vi "SOL Instruments Camera.vi"() -> ()   [LabVIEW 2015]
doc: "Example VI that demonstrates all library features."
uses:
  PL SOL Instruments Camera.lvclass
panel:
  in  "port":u16=17017
  in  "address":string="192.168.240.181"
  out "SOL Camera":refnum<class "PL SOL Instruments Camera.lvclass">
  out "error":errorcluster
  in  "stop":bool
  in  "Tab Control":enum32{"Main", "Parameters", "Info"}(tab)
  out "graph":u16[](graph)
  in  "run once":bool
  in  "run":bool
  in  "offset":dbl=-30.59628543499511 format="%#_3g"
  in  "gain":dbl=1.6 format="%#_3g"
  in  "camera parameters":T1={"number of regions"=1, "readout rate, kHz"=1000, "actual readout rate, kHz"=0, "bits per pixel"=4, "synchronization mode"=0, "OUT1 mode"=0, "OUT2 mode"=0, "exposure time, s"=0.001, "delay before exposure, s"=1e-06, "delay after exposure, s"=1e-06, "delay between exposures, s"=1e-06, "CCD mode"=2, "CCD advanced mode"=0, "X read mode"=0, "Y read mode"=1, "prechanrge bus"=0, "options"={"x averaging"=FALSE, "x subsampling"=FALSE, "y subsampling"=FALSE, "y averaging"=FALSE}, "nondestructive frame delays, s"=[1e-06, 1e-06, 1e-06, 1e-06, 1e-06, 1e-06, 1e-06, 1e-06], "double slope reset time, s"=1e-06, "DAC"=32, "gamma correction"=0} {"double slope reset time, s" format="%#_6p"; "nondestructive frame delays, s" format="%#_3p"; "prechanrge bus" items=["no", "yes"]; "Y read mode" items=["forward", "backward"]; "X read mode" items=["forward", "backward"]; "CCD advanced mode" items=["none", "nondestructive", "double slope"]; "CCD mode" items=["parallel", "serial", "low dark current", "large full well"]; "delay between exposures, s" format="%#_3p"; "delay after exposure, s" format="%#_3p"; "delay before exposure, s" format="%#_3p"; "exposure time, s" format="%#_3p"; "OUT2 mode" items=["exposure (negative)", "exposure (positive)", "delay before esposure (negative)", "delay after esposure (negative)", "external input inverted", "external input", "user register bit 1", "software start scan", "reserved"]; "OUT1 mode" items=["exposure (negative)", "exposure (positive)", "delay before esposure (negative)", "delay after esposure (negative)", "external input inverted", "external input", "user register bit 0", "software start scan", "reserved"]; "synchronization mode" items=["software"=0, "hardware"=1, "external rising edge type 1"=2, "external rising edge type 2"=3, "external falling edge type 1"=10, "external falling edge type 2"=11]; "readout rate, kHz" items=["1000"=1000, "500"=500, "250"=250, "125"=125]; "bits per pixel" items=["8", "10", "12", "14", "16"]}
  out "regions":T2(array[cluster])
  out "controller info":T3
  out "camera info":T4 {"sensor type" items=["unknown"=0, "S9840"=1, "S7017-1007"=10, "S7017-1008"=11, "S7030-0908"=20, "S7030-1006"=21, "S7030-1008"=22, "S7031-1006"=30, "S7031-1007"=31, "S7031-1008"=32, "S7170-0909"=40, "S7171-0909"=41, "S7172-0909"=42, "S8378-1024Q"=50, "S8667-1010"=51, "S9737-01"=60, "S9970-1007"=70, "S10141-1109"=80, "S10142-1107"=90, "S10142-1108"=91, "S10142-1109"=92, "G9201-256S"=100, "G9202-512S"=101, "G9203-256S"=102, "G9204-512S"=103, "G9208-256W"=104, "I5-A1300-M2"=110, "I5-A1300-C2"=111, "LUPA-4000M"=200]; "delay between exposures"."min, s" format="%#_6p"; "delay after exposure"."min, s" format="%#_6p"; "delay before exposure"."min, s" format="%#_6p"; "exposure time"."min, s" format="%#_6p"; "cooling"."type" items=["no sensors", "3 sensors", "1 sensor"]}
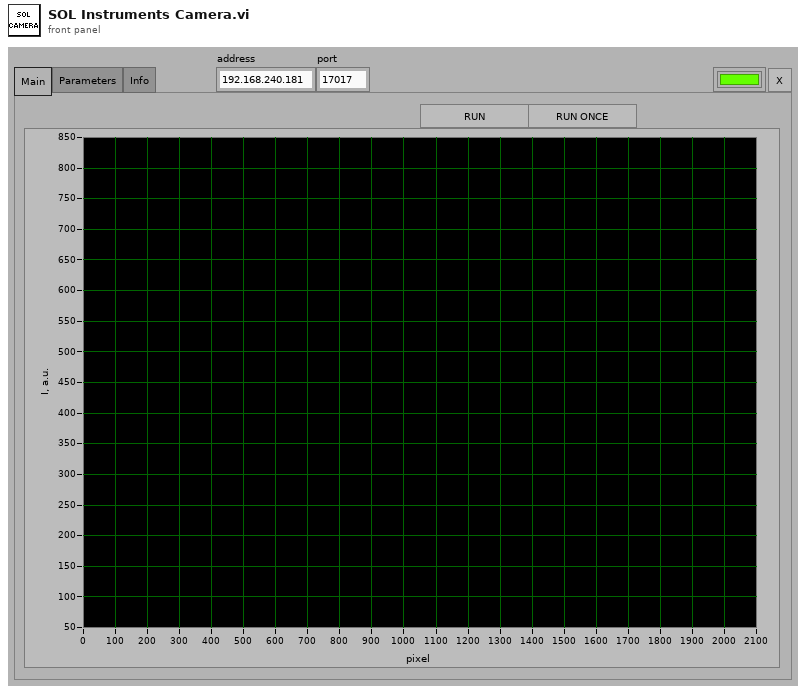
[diagram p1: front panel]
types:
  T1 = cluster{"number of regions":i32, "readout rate, kHz":i32, "actual readout rate, kHz":i32, "bits per pixel":u16, "synchronization mode":u16, "OUT1 mode":u16, "OUT2 mode":u16, "exposure time, s":dbl, "delay before exposure, s":dbl, "delay after exposure, s":dbl, "delay between exposures, s":dbl, "CCD mode":u16, "CCD advanced mode":u16, "X read mode":u16, "Y read mode":u16, "prechanrge bus":u16, "options":cluster{"x averaging":bool, "x subsampling":bool, "y subsampling":bool, "y averaging":bool}, "nondestructive frame delays, s":dbl[], "double slope reset time, s":dbl, "DAC":u16, "gamma correction":u16}
  T2 = cluster{"left":u16, "top":u16, "right":u16, "bottom":u16, "region number":u16, "super pixel height":u16, "super pixel width":u16}[]
  T3 = cluster{"memory size, MB":i32, "os":string, "software version":string, "FPGA version":string, "device name":string, "serial number":string}
  T4 = cluster{"frame":cluster{"width":u16, "height":u16}, "cooling":cluster{"type":u16, "temperature range":cluster{"min":i32, "max":i32}}, "frame rates, kHz":i32[], "pixel":cluster{"width, mkm":dbl, "height. mkm":dbl}, "max binning":cluster{"horizontal":u16, "vertical":u16}, "max number of regions":u16, "region size constraints":cluster{"even start":bool, "div by 4":bool, "div by 8":bool, "div by 16":bool, "fvb only":bool, "width":cluster{"min":u16, "max":u16}, "height":cluster{"min":u16, "max":u16}}, "number of fans":u16, "RAM":cluster{"size, MB":u16, "max number of frames":u32}, "number of outputs":u16, "number of synchronization modes":u16, "number of OUT1 modes":u16, "number of OUT2 modes":u16, "exposure time":cluster{"min, s":dbl, "max, s":dbl}, "delay before exposure":cluster{"min, s":dbl, "max, s":dbl}, "delay after exposure":cluster{"min, s":dbl, "max, s":dbl}, "delay between exposures":cluster{"min, s":dbl, "max, s":dbl}, "sensor type":u16}
  T5 = cluster{"frame":cluster{"width":u16, "height":u16}, "cooling":cluster{"type":u16, "temperature range":cluster{"min":i32, "max":i32}}, "readout rates, kHz":i32[], "pixel":cluster{"width, mkm":dbl, "height. mkm":dbl}, "max binning":cluster{"horizontal":u16, "vertical":u16}, "max number of regions":u16, "region size constraints":cluster{"even start":bool, "div by 4":bool, "div by 8":bool, "div by 16":bool, "fvb only":bool, "width":cluster{"min":u16, "max":u16}, "height":cluster{"min":u16, "max":u16}}, "number of fans":u16, "RAM":cluster{"size, MB":u16, "max number of frames":u32}, "number of outputs":u16, "number of synchronization modes":u16, "number of OUT1 modes":u16, "number of OUT2 modes":u16, "exposure time":cluster{"min, us":dbl, "max, s":dbl}, "delay before exposure":cluster{"min, s":dbl, "max, s":dbl}, "delay after exposure":cluster{"min, s":dbl, "max, s":dbl}, "delay between exposures":cluster{"min, s":dbl, "max, s":dbl}, "sensor type":u16}
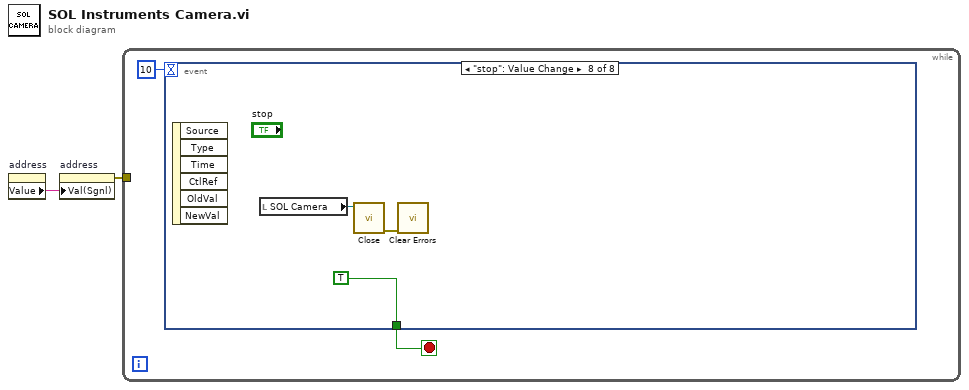
[diagram p0: block diagram]
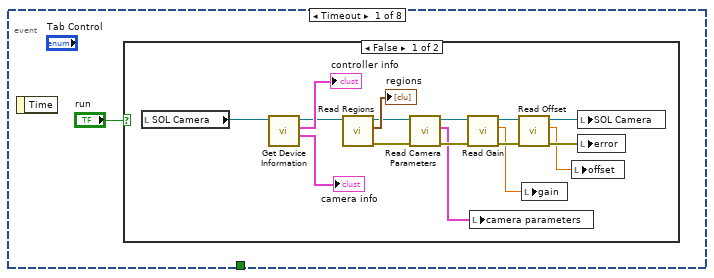
[diagram p2: hidden frame]
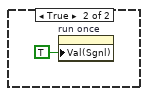
[diagram p3: hidden frame]
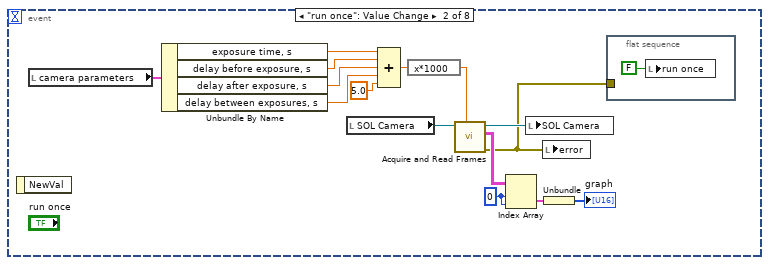
[diagram p4: hidden frame]
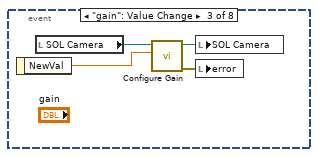
[diagram p5: hidden frame]
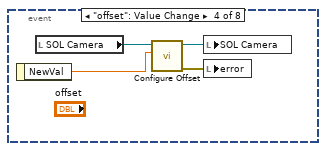
[diagram p6: hidden frame]
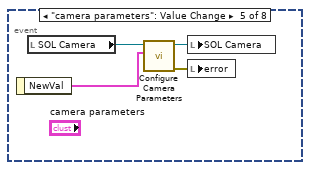
[diagram p7: hidden frame]
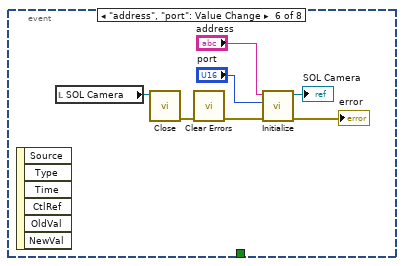
[diagram p8: hidden frame]
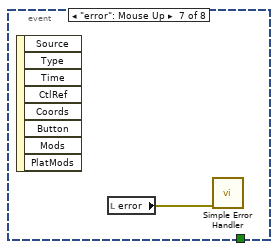
[diagram p9: hidden frame]
diagram:
  n1 = property on="address" class="Str"() -> ("Value"=w2:string)  [unwired: 2 in, 2 out]
  n2 = property on="address" class="Str"("Val(Sgnl)"=w2) -> (error out=w1:errorcluster)  [unwired: 2 in, 1 out]
  n3 = while {
    tunnel: w1 -> [_]
    stop <- w4 stop-if-true
    n4 = event shown="[7] \"stop\": Value Change" {
      selector: _ -> [_ _ _ _ _ _ _ _]
      dyn-events: _ -> [_ _ _ _ _ _ _ _]
      timeout: 10 -> [_ _ _ _ _ _ _ _]
      tunnel: [_ _ _ _ _ _ _ TRUE ("stop")] -> w4
      event Timeout {
        n5 = event-data() -> ()  [unwired: 1 in, 1 out]
        n6 = case shown="False" "run" {
          frame False {
            n7 = local read "SOL Camera"() -> (w17:refnum<class "PL SOL Instruments Camera.lvclass">)
            n8 = call "Get Device Information.vi"("SOL Camera in"=w17) -> ("camera information"=→"camera info":T5, "controller information"=→"controller info":T3, "SOL Camera out"=w18:refnum<class "PL SOL Instruments Camera.lvclass">)  [unwired: 8 in]
            n9 = call "Read Regions.vi"("SOL Camera in"=w18) -> ("error out"=w15:errorcluster, "regions"=→"regions":T2, "SOL Camera out"=w16:refnum<class "PL SOL Instruments Camera.lvclass">)  [unwired: 8 in]
            n10 = call "Read Camera Parameters.vi"("error in (no error)"=w15, "SOL Camera in"=w16) -> ("error out"=w11:errorcluster, "parameters"=w8:T1, "SOL Camera out"=w14:refnum<class "PL SOL Instruments Camera.lvclass">)  [unwired: 7 in]
            n11 = call "Read Gain.vi"("error in (no error)"=w11, "SOL Camera in"=w14) -> ("error out"=w10:errorcluster, "gain"=w7:dbl, "SOL Camera out"=w13:refnum<class "PL SOL Instruments Camera.lvclass">)  [unwired: 7 in]
            n12 = local write "camera parameters"(w8) -> ()
            n13 = call "Read Offset.vi"("error in (no error)"=w10, "SOL Camera in"=w13) -> ("error out"=w9:errorcluster, "offset"=w6:dbl, "SOL Camera out"=w12:refnum<class "PL SOL Instruments Camera.lvclass">)  [unwired: 7 in]
            n14 = local write "gain"(w7) -> ()
            n15 = local write "offset"(w6) -> ()
            n16 = local write "SOL Camera"(w12) -> ()
            n17 = local write "error"(w9) -> ()
          }
          frame True {
            n18 = property on="run once" class="Bool (strict)"("Val(Sgnl)"=TRUE ("Value (Signaling)")) -> ()  [unwired: 2 in, 2 out]
          }
        }
      }
      event "run once": Value Change {
        w24 = 0 ("index (row)")
        n19 = event-data() -> ()  [unwired: 1 in, 1 out]
        n20 = local read "camera parameters"() -> (w32:T1)
        n21 = Unbundle By Name(w32) -> ("exposure time, s"=w31:dbl, "delay before exposure, s"=w30:dbl, "delay after exposure, s"=w29:dbl, "delay between exposures, s"=w28:dbl)
        n22 = local read "SOL Camera"() -> (w33:refnum<class "PL SOL Instruments Camera.lvclass">)
        n23 = Compound Arithmetic op=ADD(w31, w30, w29, w28, 5.0 ("value")) -> (w26:dbl)
        n24 = expression code="x*1000"(w26) -> (w25:dbl)
        n25 = call "Acquire and Read Frames.vi"("additional timeout, ms (0)"=w25, "SOL Camera in"=w33) -> ("error out"=w34:errorcluster, "frames"=w36:cluster{u16[]}[][], "SOL Camera out"=w37:refnum<class "PL SOL Instruments Camera.lvclass">)  [unwired: 7 in]
        n26 = Index Array(array=w36, index (row)=w24, index (col)=w24) -> (element=w35:cluster{u16[]})
        n27 = local write "SOL Camera"(w37) -> ()
        n28 = local write "error"(w34) -> ()
        n29 = Unbundle(w35) -> (→"graph":u16[])
        n30 = flat-sequence {
          tunnel: w34 -> [_]
          frame #0 {
            n31 = local write "run once"(FALSE ("run once")) -> ()
          }
        }
      }
      event "gain": Value Change {
        n32 = event-data() -> ("NewVal"=w39:dbl)  [unwired: 1 in]
        n33 = local read "SOL Camera"() -> (w42:refnum<class "PL SOL Instruments Camera.lvclass">)
        n34 = call "Configure Gain.vi"("gain"=w39, "SOL Camera in"=w42) -> ("error out"=w40:errorcluster, "SOL Camera out"=w41:refnum<class "PL SOL Instruments Camera.lvclass">)  [unwired: 8 in]
        n35 = local write "SOL Camera"(w41) -> ()
        n36 = local write "error"(w40) -> ()
      }
      event "offset": Value Change {
        n37 = event-data() -> ("NewVal"=w43:dbl)  [unwired: 1 in]
        n38 = local read "SOL Camera"() -> (w46:refnum<class "PL SOL Instruments Camera.lvclass">)
        n39 = call "Configure Offset.vi"("offset"=w43, "SOL Camera in"=w46) -> ("error out"=w44:errorcluster, "SOL Camera out"=w45:refnum<class "PL SOL Instruments Camera.lvclass">)  [unwired: 8 in]
        n40 = local write "SOL Camera"(w45) -> ()
        n41 = local write "error"(w44) -> ()
      }
      event "camera parameters": Value Change {
        n42 = event-data() -> ("NewVal"=w48:T1)  [unwired: 1 in]
        n43 = local read "SOL Camera"() -> (w50:refnum<class "PL SOL Instruments Camera.lvclass">)
        n44 = call "Configure Camera Parameters.vi"("parameters"=w48, "SOL Camera in"=w50) -> ("error out"=w47:errorcluster, "SOL Camera out"=w49:refnum<class "PL SOL Instruments Camera.lvclass">)  [unwired: 8 in]
        n45 = local write "SOL Camera"(w49) -> ()
        n46 = local write "error"(w47) -> ()
      }
      event "address", "port": Value Change {
        n47 = event-data() -> ()  [unwired: 1 in, 6 out]
        n48 = local read "SOL Camera"() -> (w56:refnum<class "PL SOL Instruments Camera.lvclass">)
        n49 = call "Close.vi"("SOL Camera in"=w56) -> ("error out"=w57:errorcluster)  [unwired: 10 in]
        n50 = call <vilib>:"Clear Errors.vi"("error in (no error)"=w57) -> ("error out"=w54:errorcluster)  [unwired: 5 in, 1 out]
        n51 = call "Initialize.vi"("error in (no error)"=w54, "port (17017)"="port", "address (192.168.240.181)"="address") -> ("error out"=→"error":errorcluster, "SOL Camera out"=→"SOL Camera":refnum<class "PL SOL Instruments Camera.lvclass">)  [unwired: 7 in]
      }
      event "error": Mouse Up {
        n52 = event-data() -> ()  [unwired: 1 in, 8 out]
        n53 = local read "error"() -> (w58:errorcluster)
        n54 = call <vilib>:"Simple Error Handler.vi"("error in (no error)"=w58) -> ()  [unwired: 4 in, 5 out]
      }
      event "stop": Value Change {
        n55 = event-data() -> ()  [unwired: 1 in, 6 out]
        n56 = local read "SOL Camera"() -> (w59:refnum<class "PL SOL Instruments Camera.lvclass">)
        n57 = call "Close.vi"("SOL Camera in"=w59) -> ("error out"=w60:errorcluster)  [unwired: 10 in]
        n58 = call <vilib>:"Clear Errors.vi"("error in (no error)"=w60) -> ()  [unwired: 5 in, 2 out]
      }
    }
  }
